vi "Write Cumulative_mean_square .vi"(8 "error in (no error)":errorcluster, 10 "Cumulative_mean_square":dbl, 11 "Online_Statistic in":refnum<class "Online_Statistic.lvclass">) -> (0 "error out":errorcluster, 3 "Online_Statistic out":refnum<class "Online_Statistic.lvclass">)   [LabVIEW 2021, in "Online_Statistic.lvclass"]
uses:
  Online_Statistic.lvclass
  Online_Statistic.lvclass/Online_Statistic.ctl
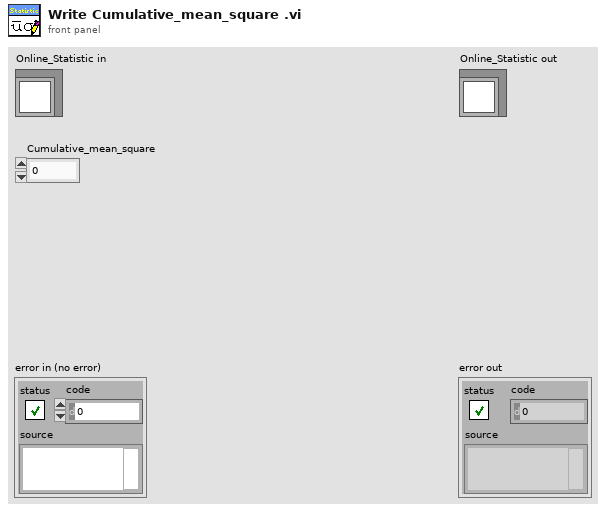
[diagram p1: front panel]
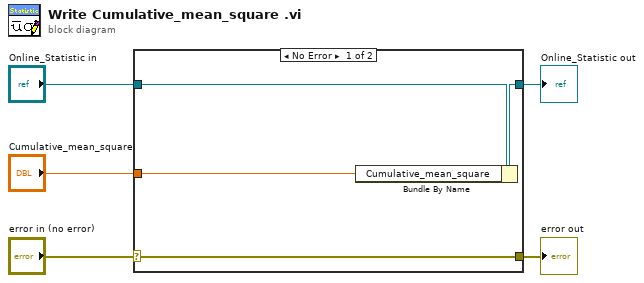
[diagram p0: block diagram]
diagram:
  n1 = case shown="No Error" "error in (no error)" {
    selector: "error in (no error)" -> [w9 w10]
    tunnel: [w9 w10] -> w4
    tunnel: [w7 w11] -> w2
    tunnel: "Online_Statistic in" -> [w8 w11]
    tunnel: "Cumulative_mean_square" -> [w6 _]
    frame No Error {
      n2 = Bundle By Name(cluster=w8, "Cumulative_mean_square"=w6) -> (w7:refnum<class "Online_Statistic.lvclass">)
    }
    frame Error {
    }
  }
  "error out" <- w4
  "Online_Statistic out" <- w2
